vi "gyro -- launch async fitter.vi"(11 "fitter pair":T1) -> (2 "reference out":refnum<vi>, 3 "fitter pair OUT":T1)   [LabVIEW 2018]
uses:
  server talk-to-back pair.ctl
  server talkback message type.ctl
  server talkto message type.ctl
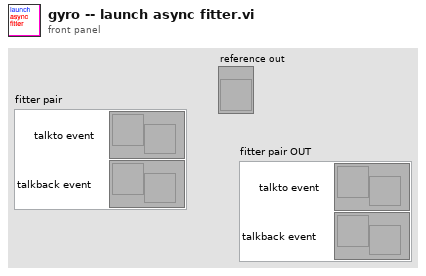
[diagram p1: front panel]
types:
  T1 = typedef "server talk-to-back pair.ctl" = cluster{"talkback event":refnum<user-event>, "talkto event":refnum<user-event>}
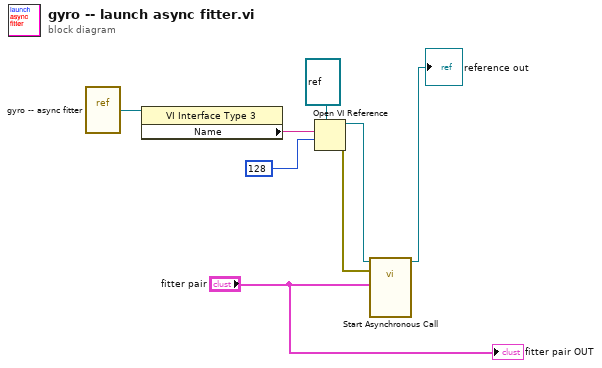
[diagram p0: block diagram]
diagram:
  n1 = vi-ref "gyro -- async fitter.vi"() -> (w7:refnum<vi>)
  n2 = property class="VI Interface Type 3"(reference=w7) -> ("Name"=w6:string)  [unwired: 1 in, 2 out]
  n3 = Open VI Reference(type specifier VI Refnum (for type only)=refnum<vi> refnum, vi path=w6, options=128) -> (vi reference=w3:refnum<vi>, error out=w2:errorcluster)  [unwired: 3 in]
  n4 = call-by-ref "Start Asynchronous Call"(reference=w3, error in=w2, "pll event pair"="fitter pair") -> (reference out=→"reference out":refnum<vi>)  [unwired: 11 in, 1 out]
  "fitter pair OUT" <- "fitter pair"
